vi "Close Registry Key.vi"(4 "error in (no error)":errorcluster, 7 "refnum":T1) -> (0 "error out":errorcluster)   [LabVIEW 2020]
doc: "Closes a key in the Windows registry."
uses:
  Registry refnum.ctl
  Advapi32.dll
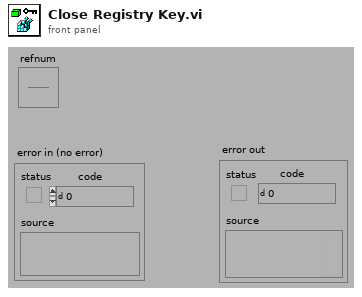
[diagram p1: front panel]
types:
  T1 = typedef "Registry refnum.ctl" = refnum<k1>
  T2 = enum16{"store handles", "dispose handles", "get handles"}
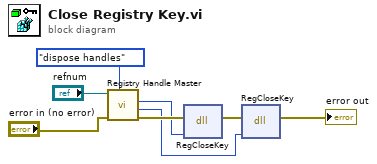
[diagram p0: block diagram]
diagram:
  n1 = call "Registry Handle Master.vi"("action (get handles)"=T2."dispose handles", "error in (no error)"="error in (no error)", "refnum"="refnum") -> ("error out"=w5:errorcluster, "remote key handle out"=w3:u64, "key handle out"=w4:u64)  [unwired: 3 in, 3 out]
  n2 = dll-call lib="Advapi32.dll" fn="RegCloseKey"(error in=w5, "phk"=w4) -> (error out=w2:errorcluster)  [unwired: 3 in, 2 out]
  n3 = dll-call lib="Advapi32.dll" fn="RegCloseKey"(error in=w2, "phk"=w3) -> (error out=→"error out":errorcluster)  [unwired: 3 in, 2 out]
